vi "Disconnect LTS Stage.vi"(8 "error in (no error)":errorcluster, 10 "Cluster in":T1, 11 "LTS Reference In":refnum<k24>) -> (0 "error out":errorcluster, 2 "Cluster out":T1, 3 "LTS Reference Out":refnum<k24>)   [LabVIEW 2018]
uses:
  Controls/Translation Stage Cluster.ctl
  General/Controls/Translation Stage Types.ctl
  C:/Project/SerialSectOCT/SerialSectOCT/Software/Thorlabs.MotionControl.Controls.dll
  Thorlabs.MotionControl.Controls.dll
panel:
  out "CloseDevice":bool
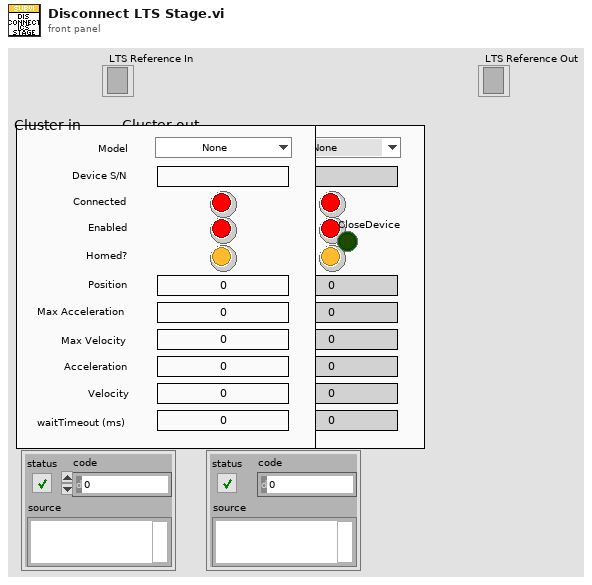
[diagram p1: front panel]
types:
  T1 = typedef "Translation Stage Cluster.ctl" = cluster{"Position":dbl, "Is.Enabled?":bool, "Is.Connected?":bool, "Device SN":string, "AccelerationMaximum":dbl, "VelocityMaximum":dbl, "Acceleration":dbl, "Velocity":dbl, "waitTimeout (ms)":i32, "Model":T2, "Is.Homed?":bool}
  T2 = typedef "Translation Stage Types.ctl" = enum16{"None", "Thorlabs LTS", "Thorlabs MLJ"}
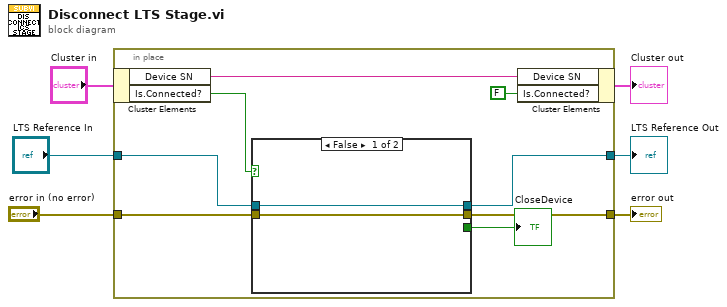
[diagram p0: block diagram]
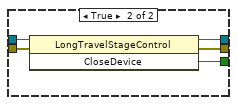
[diagram p2: hidden frame]
diagram:
  n1 = in-place {
    in-place-border: "LTS Reference In" -> [w12]
    in-place-border: "error in (no error)" -> [w10]
    in-place-border: [w11] -> w2
    in-place-border: [w9] -> w1
    n2 = in-place-cluster #1("Cluster in") -> ("Device SN"=w14:string, "Is.Connected?"=w7:bool)
    n3 = case shown="False" w7 {
      tunnel: w12 -> [w15 w21]
      tunnel: [w15 w20] -> w11
      tunnel: w10 -> [w16 w19]
      tunnel: [w16 w18] -> w9
      tunnel: [_ w17] -> w8
      frame False {
      }
      frame True {
        n4 = invoke class="LongTravelStageControl" method="CloseDevice"(reference=w21, error in=w19) -> (reference out=w20:refnum<k24>, error out=w18:errorcluster, "CloseDevice"=w17:bool)  [unwired: 1 in]
      }
    }
    "CloseDevice" <- w8
    n5 = in-place-cluster #1("Device SN"=w14, "Is.Connected?"=FALSE) -> (→"Cluster out":T1)
  }
  "error out" <- w1
  "LTS Reference Out" <- w2
